vi "PI_controller.vi"(8 "absolute":dbl format="%#_4g", 10 "desired":dbl) -> (1 "degree error":dbl format="%#.3g", 2 "direction":dbl, 5 "step size":i32)   [LabVIEW 2020]
panel:
  out "position error":dbl
  out "step error":dbl format="%#.3f"
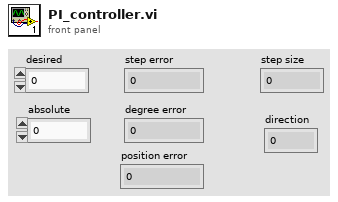
[diagram p1: front panel]
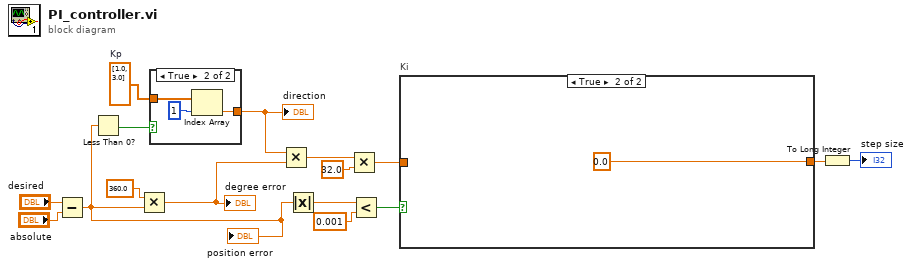
[diagram p0: block diagram]
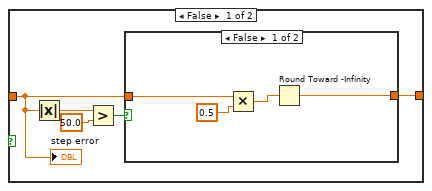
[diagram p2: hidden frame]
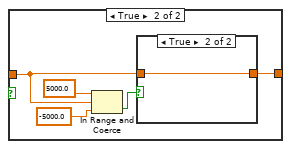
[diagram p3: hidden frame]
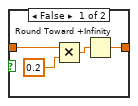
[diagram p4: hidden frame]
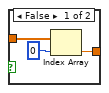
[diagram p5: hidden frame]
diagram:
  w14 = dbl[] [1.0, 3.0]  # Kp
  n1 = Subtract ("error")(x="desired", y="absolute") -> (x-y=w2:dbl)
  "position error" <- w2
  n2 = Less Than 0?(x=w2) -> (x < 0?=w13:bool)
  n3 = Multiply(x=360.0, y=w2) -> (x*y=w3:dbl)
  "degree error" <- w3
  n4 = case shown="True" w13 {
    tunnel: [w18 w20] -> w16
    tunnel: w14 -> [w19 w22]
    frame False {
      n5 = Index Array(array=w19, index=0) -> (element=w18:dbl)
    }
    frame True {
      n6 = Index Array(array=w22, index=1) -> (element=w20:dbl)
    }
  }
  "direction" <- w16
  n7 = Multiply(x=w16, y=w3) -> (x*y=w10:dbl)
  n8 = Absolute Value(x=w2) -> (abs(x)=w6:dbl)
  n9 = Multiply(x=w10, y=32.0) -> (x*y=w12:dbl)
  n10 = Less?(x=w6, y=0.001) -> (x < y?=w9:bool)
  n11 = case "Ki" shown="True" w9 {
    tunnel: [w27 0.0] -> w1
    tunnel: w12 -> [w23 _]
    frame False {
      n12 = Absolute Value(x=w23) -> (abs(x)=w26:dbl)
      n13 = Greater?(x=w26, y=50.0) -> (0:w24:bool)
      n14 = case shown="False" w24 {
        tunnel: [w28 w36] -> w27
        tunnel: w23 -> [w30 w34]
        frame False {
          n15 = Multiply(x=w30, y=0.5) -> (x*y=w29:dbl)
          n16 = Round Toward -Infinity(1:w29) -> (0:w28:dbl)
        }
        frame True {
          n17 = In Range and Coerce(upper limit=5000.0 ("high step"), x=w34, lower limit=-5000.0 ("low step")) -> (In Range?=w32:bool)  [unwired: 1 out]
          n18 = case shown="True" w32 {
            tunnel: [w37 w41] -> w36
            tunnel: w34 -> [w39 w41]
            frame False {
              n19 = Multiply(x=w39, y=0.2) -> (x*y=w38:dbl)
              n20 = Round Toward +Infinity(x=w38) -> (ceil(x): smallest int >= x=w37:dbl)
            }
            frame True {
            }
          }
        }
      }
      "step error" <- w23
    }
    frame True {
    }
  }
  n21 = To Long Integer(number=w1) -> (32bit integer=→"step size":i32)
